vi "create.SequencedUnitHeader.vi"(8 "error in (no error)":errorcluster, 10 "SequencedUnitHeader.Parms":T1={"Hdr Count"=0, "Hdr Unit"=0, "Hdr Sequence"=1, "Starting Sequence"=1}, 11 "SequencedUnitHeader in":refnum<class "SequencedUnitHeader.lvclass">) -> (0 "error out":errorcluster, 3 "SequencedUnitHeader out":refnum<class "SequencedUnitHeader.lvclass">)   [LabVIEW 2020, in "SequencedUnitHeader.lvclass"]
uses:
  SequencedUnitHeader.lvclass
  SequencedUnitHeader.Parameters.ctl
  FieldSpec.ctl
  SequencedUnitHeader.lvclass/SequencedUnitHeader.ctl
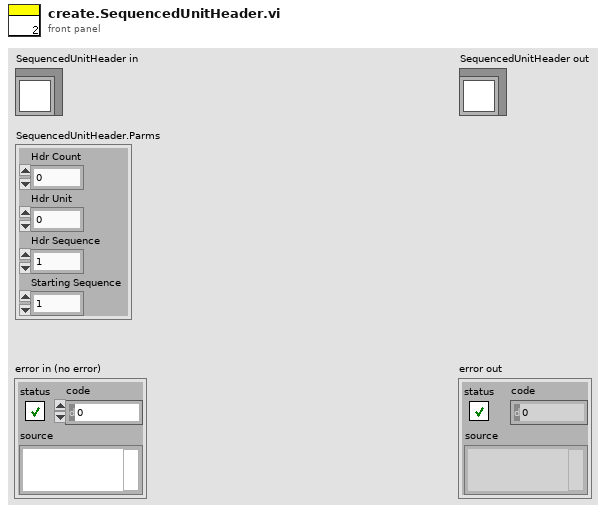
[diagram p1: front panel]
types:
  T1 = typedef "SequencedUnitHeader.lvclass/SequencedUnitHeader.Parameters.ctl" = cluster{"Hdr Count":u8, "Hdr Unit":u8, "Hdr Sequence":u32, "Starting Sequence":u32}
  T2 = typedef "FieldSpec.ctl" = cluster{"Name":string, "Offset":i32, "Length":i32, "FieldType":enum16{"Alphanumeric", "Binary", "BinaryLongPrice", "BinaryShortPrice", "BitField", "PrintableAscii", "Value"}, "FieldValue":variant}
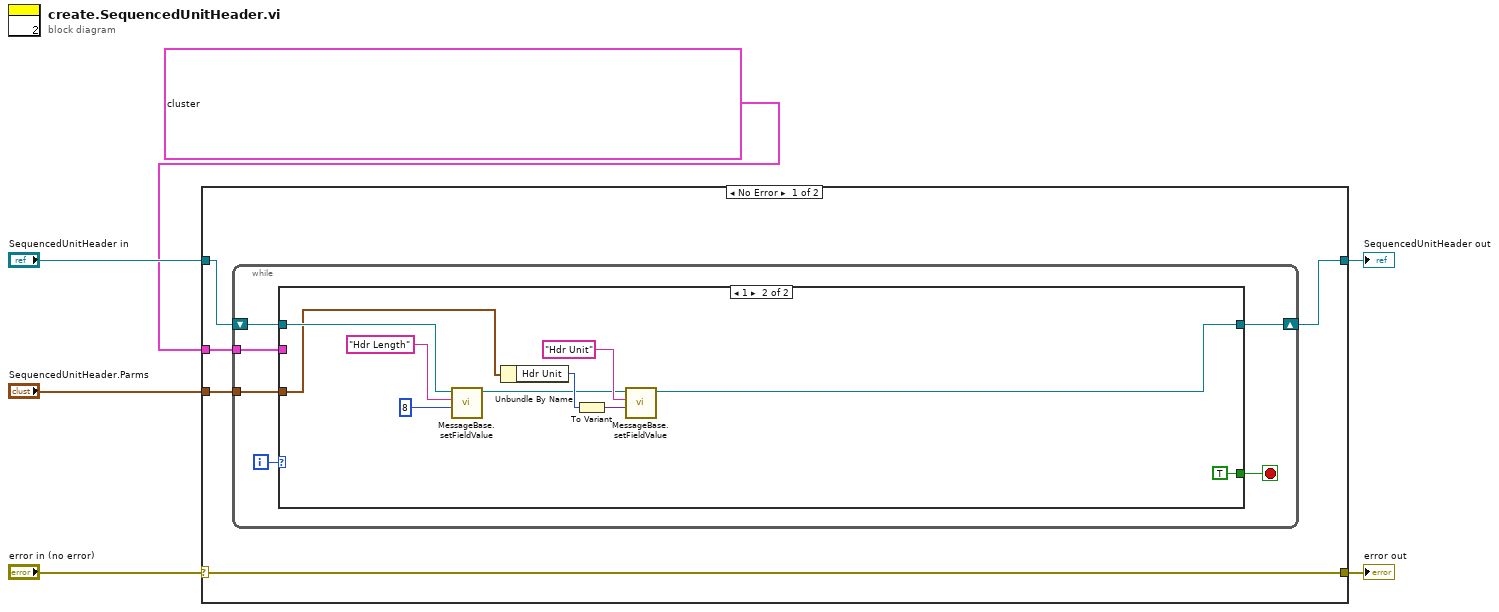
[diagram p0: block diagram]
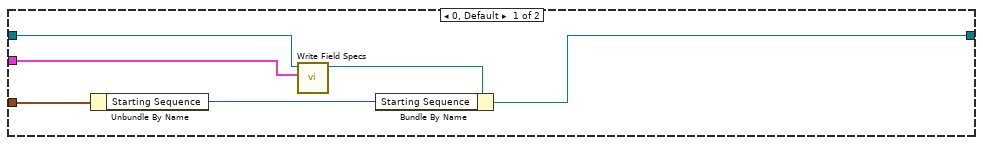
[diagram p2: hidden frame]
diagram:
  n1 = case shown="No Error" "error in (no error)" {
    selector: "error in (no error)" -> [w11 w35]
    tunnel: [w11 w35] -> w5
    tunnel: [w7 w34] -> w3
    tunnel: "SequencedUnitHeader in" -> [w8 w34]
    tunnel: T2[] [{"Name"="Hdr Length", "Offset"=0, "Length"=2, "FieldType"=enum."Binary", "FieldValue"=variant}, {"Name"="Hdr Count", "Offset"=2, "Length"=1, "FieldType"=enum."Binary", "FieldValue"=variant}, {"Name"="Hdr Unit", "Offset"=3, "Length"=1, "FieldType"=enum."Binary", "FieldValue"=variant}, {"Name"="Hdr Sequence", "Offset"=4, "Length"=4, "FieldType"=enum."Binary", "FieldValue"=variant}] ("appended array") -> [w10 _]
    tunnel: "SequencedUnitHeader.Parms" -> [w9 _]
    frame No Error {
      n2 = while {
        tunnel: w10 -> [w16]
        shift-right: [w14] -> w7
        shift-left: w8 -> [w15]
        tunnel: w9 -> [w12]
        i -> [w17]
        stop <- w13 stop-if-true
        n3 = case shown="1" w17 {
          tunnel: [_ TRUE] -> w13
          tunnel: w16 -> [w23 _]
          tunnel: w15 -> [w22 w31]
          tunnel: [w18 w24] -> w14
          tunnel: w12 -> [w20 w26]
          frame 0, Default {
            n4 = Unbundle By Name(w20) -> ("Starting Sequence"=w19:u32)
            n5 = call-dynamic "Write Field Specs.vi"("Field Specs"=w23, "MessageBase in"=w22) -> ("MessageBase out"=w21:refnum<class "SequencedUnitHeader.lvclass">)  [unwired: 8 in, 1 out]
            n6 = Bundle By Name(cluster=w21, "Starting Sequence"=w19) -> (w18:refnum<class "SequencedUnitHeader.lvclass">)
          }
          frame 1 {
            n7 = call-dynamic "MessageBase.setFieldValue.vi"("Value"=u16 8, "FIeld.Name"="Hdr Length", "MessageBase in"=w31) -> ("MessageBase out"=w25:refnum<class "SequencedUnitHeader.lvclass">)  [unwired: 7 in, 1 out]
            n8 = Unbundle By Name(w26) -> ("Hdr Unit"=w33:u8)
            n9 = To Variant(anything=w33) -> (Variant=w28:variant)
            n10 = call-dynamic "MessageBase.setFieldValue.vi"("Value"=w28, "FIeld.Name"="Hdr Unit", "MessageBase in"=w25) -> ("MessageBase out"=w24:refnum<class "SequencedUnitHeader.lvclass">)  [unwired: 7 in, 1 out]
          }
        }
      }
    }
    frame Error {
    }
  }
  "error out" <- w5
  "SequencedUnitHeader out" <- w3
